vi "Lab.05_DAQ_3.vi"() -> ()   [LabVIEW 2016]
uses:
  <vilib>/Analysis/NI_AAL_SigProc.lvlib
panel:
  out "Percentage":dbl
  out "one period signal":dbl[](graph)
  out "Numeric":dbl
  out "period":dbl
  out "valleys":dbl
  out "peaks":dbl
  out "Min":dbl
  out "Max":dbl
  out "peak to peak amplitude":dbl
  out "added signal":dynamicdata(graph)
  out "input signals":dynamicdata(graph)
  in  "stop":bool
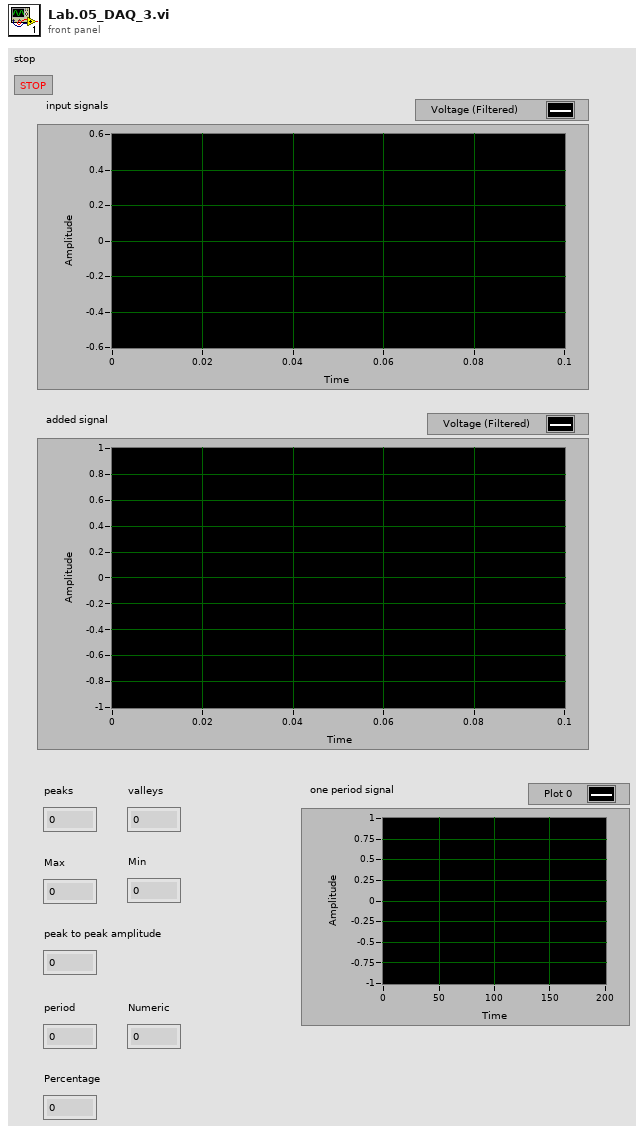
[diagram p1: front panel]
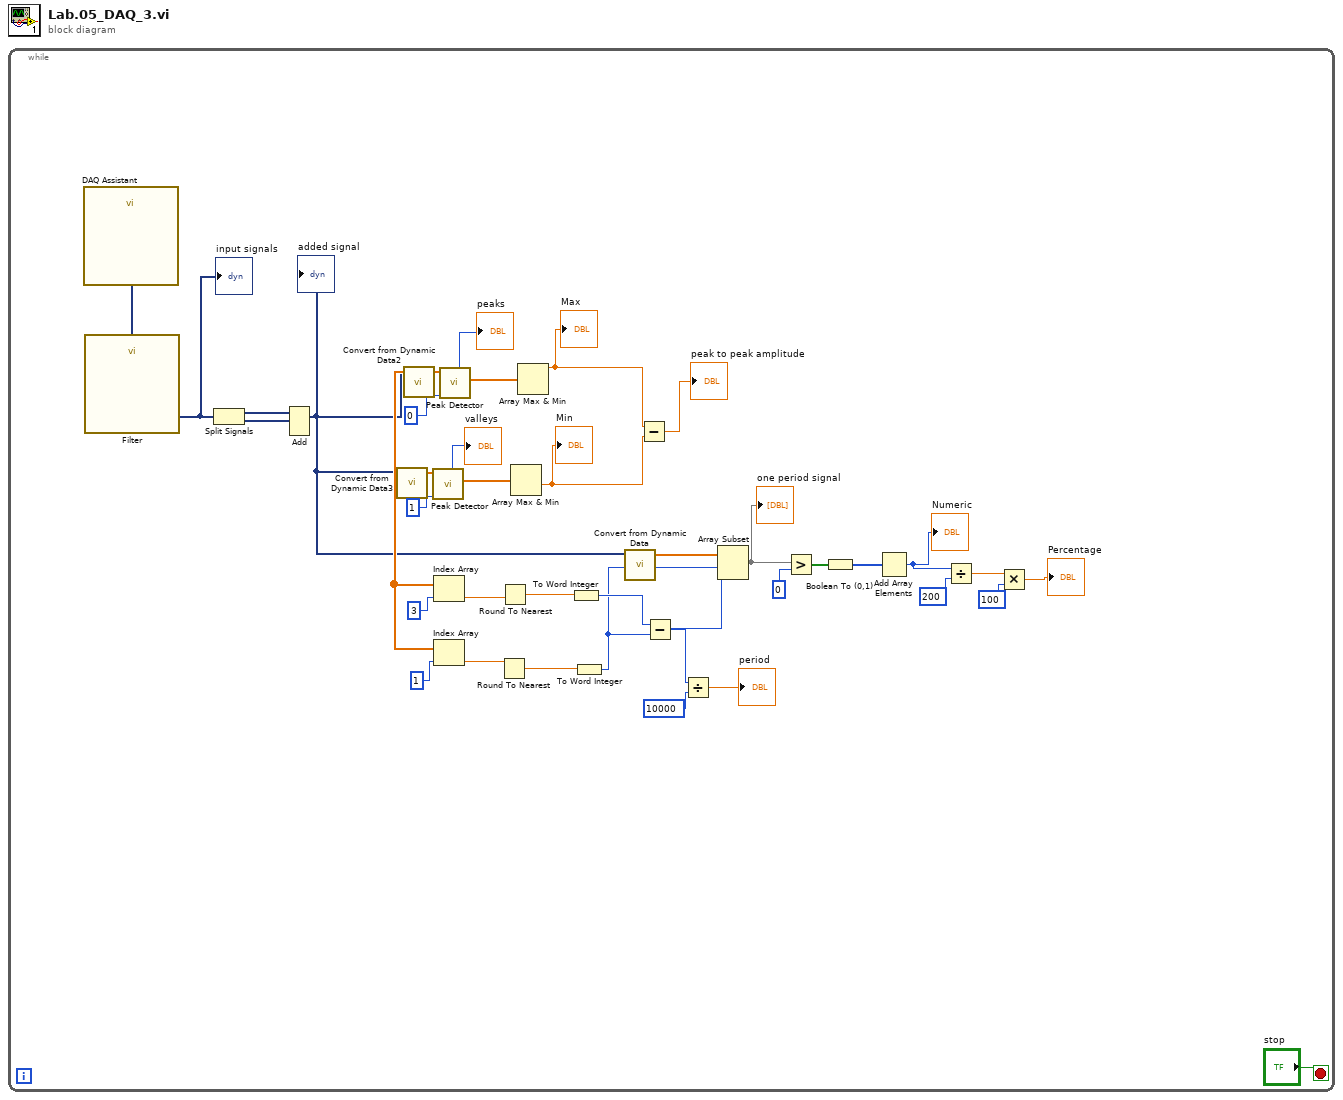
[diagram p0: block diagram]
diagram:
  n1 = while {
    stop <- "stop" stop-if-true
    n2 = call "DAQ Assistant"() -> ("data"=w38:dynamicdata)  [unwired: 16 in, 3 out]
    n3 = call "Filter"("Signal"=w38) -> ("Filtered Signal"=w29:dynamicdata)  [unwired: 9 in, 1 out]
    "input signals" <- w29
    n4 = Split Signals(w29) -> (w31:dynamicdata, w30:dynamicdata)  [unwired: 2 in]
    n5 = Add(1:w30, 2:w31) -> (0:w14:dynamicdata)  [unwired: 1 in, 1 out]
    "added signal" <- w14
    n6 = call "Convert from Dynamic Data3"("Dynamic Data Type"=w14) -> ("Array"=w35:dbl[])  [unwired: 3 in]
    n7 = call "Convert from Dynamic Data2"("Dynamic Data Type"=w14) -> ("Array"=w37:dbl[])  [unwired: 3 in]
    n8 = call <vilib>:"Peak Detector.vi"("peaks/valleys"=1, "X"=w35) -> ("Amplitudes"=w32:dbl[], "# found"=→"valleys":i32)  [unwired: 5 in, 3 out]
    n9 = call <vilib>:"Peak Detector.vi"("peaks/valleys"=0, "X"=w37) -> ("Amplitudes"=w33:dbl[], "Locations"=w22:dbl[], "# found"=→"peaks":i32)  [unwired: 5 in, 2 out]
    n10 = Index Array(array=w22, index=3) -> (element=w18:dbl)
    n11 = Index Array(array=w22, index=1) -> (element=w20:dbl)
    n12 = Round To Nearest(number=w20) -> (nearest integer value=w19:dbl)
    n13 = Round To Nearest(number=w18) -> (nearest integer value=w17:dbl)
    n14 = Array Max & Min(array=w32) -> (min value=w28:dbl)  [unwired: 3 out]
    "Min" <- w28
    n15 = Array Max & Min(array=w33) -> (max value=w27:dbl)  [unwired: 3 out]
    "Max" <- w27
    n16 = To Word Integer(number=w17) -> (16bit integer=w16:i16)
    n17 = To Word Integer(number=w19) -> (16bit integer=w12:i16)
    n18 = call "Convert from Dynamic Data"("Dynamic Data Type"=w14) -> ("Array"=w15:dbl[])  [unwired: 3 in]
    n19 = Subtract(x=w27, y=w28) -> (x-y=→"peak to peak amplitude":dbl)
    n20 = Subtract(x=w16, y=w12) -> (x-y=w2:i16)
    n21 = Divide(x=w2, y=10000) -> (x/y=→"period":dbl)
    n22 = Array Subset(array=w15, index=w12, length=w2) -> (w9:dbl[])
    "one period signal" <- w9
    n23 = Greater?(x=w9, y=0) -> (0:w11:bool[])
    n24 = Boolean To (0,1)(Boolean=w11) -> (0, 1=w10:i16[])
    n25 = Add Array Elements(numeric array=w10) -> (sum=w7:i16)
    "Numeric" <- w7
    n26 = Divide(x=w7, y=200) -> (x/y=w5:dbl)
    n27 = Multiply(x=w5, y=100) -> (x*y=→"Percentage":dbl)
  }
